vi "GUI_OpticalSpectromete_oldr.vi"() -> ()   [LabVIEW 2009]
uses:
  shared programs/sentCommandSetting.vi
panel:
  out "new D Data":bool=TRUE
  out "new S Data":bool
  out "new Slow Data":bool=TRUE
  out "error out 5":errorcluster
  out "new Device Data":bool=TRUE
  in  "Tab Control 2":enum32{"debug", "plain", "plain 2"}(tab)
  out "message from device":string
  out "data out 2":string
  out "error out 3":errorcluster
  in  "after substring":string="-0.089798,-0.012312,-0.023161,-0.029413,-0.099722,-0.082148,-0.175780,-0.016640,-0.021793,-0.106872,-0.083723,0.034795,-0.021191,0.038109,0.089728,0.030656,0.190136,0.095931,0.069651,0.042030,-0.035811,-0.039992,-0.152535,-0.081980,-0.239391,-0.299099,-0.220282,-0.102308,-0.243030,-0.071880,-0.064330,0.057168,0.183804,0.430142,0.593920,0.668964,0.765233,0.852774,1.014855,0.897499,1.075418,0.964040,0.859461,0.844898,0.817245,0.729092,0.485039,0.430748,0.147230,0.101254,-0.023353,0.001419,-0.101078,-0.215137,-0.151236,-0.187878,-0.201514,-0.145757,-0.076726,-0.030284,0.027449,0.054593,0.122555,0.149751,0.201496,0.172129,0.177528,0.053173,0.056690,-0.060797,-0.012635,-0.050433,-0.055065,-0.118074,-0.067874,-0.150187,-0.037475,-0.162903,0.037664,-0.067378,0.033191,0.067444,0.129342,0.131002,0.036134,0.129384,0.095361,0.030507,0.046942,-0.075844,-0.066935,0.066320,-0.017437,0.050973,-0.012719,-0.028872,-0.007972,-0.092477,-0.020650,-0.016307\r\n"
  in  "command 3":string="1Darray"
  in  "after substring 3":string
  out "settings 2":string[][](array[string])=[["no error", ">>on"]]
  in  "data out 3":string="Spectrometer>>1Darray>>-0.089798,-0.012312,-0.023161,-0.029413,-0.099722,-0.082148,-0.175780,-0.016640,-0.021793,-0.106872,-0.083723,0.034795,-0.021191,0.038109,0.089728,0.030656,0.190136,0.095931,0.069651,0.042030,-0.035811,-0.039992,-0.152535,-0.081980,-0.239391,-0.299099,-0.220282,-0.102308,-0.243030,-0.071880,-0.064330,0.057168,0.183804,0.430142,0.593920,0.668964,0.765233,0.852774,1.014855,0.897499,1.075418,0.964040,0.859461,0.844898,0.817245,0.729092,0.485039,0.430748,0.147230,0.101254,-0.023353,0.001419,-0.101078,-0.215137,-0.151236,-0.187878,-0.201514,-0.145757,-0.076726,-0.030284,0.027449,0.054593,0.122555,0.149751,0.201496,0.172129,0.177528,0.053173,0.056690,-0.060797,-0.012635,-0.050433,-0.055065,-0.118074,-0.067874,-0.150187,-0.037475,-0.162903,0.037664,-0.067378,0.033191,0.067444,0.129342,0.131002,0.036134,0.129384,0.095361,0.030507,0.046942,-0.075844,-0.066935,0.066320,-0.017437,0.050973,-0.012719,-0.028872,-0.007972,-0.092477,-0.020650,-0.016307\r\n"
  out "after substring 2":string="no error,>>on"
  out "device ID":refnum<k16>
  in  "Tab Control":enum32{"Main", "Network settings", "internal"}(tab)
  in  "getSettings":bool
  in  "setTrigger":bool
  in  "String":string="subscribe>>opticalspectrometer"
  in  "sent":bool
  in  "setSave":bool
  out "save":bool
  in  "setExposure":dbl=2.0
  out "exposure out":dbl=2.0
  out "value":string
  out "trigger":bool
  out "array 2":dbl[](graph)=[-0.089798, -0.012312, -0.023161, -0.029413, -0.099722, -0.082148, -0.17578, -0.01664, -0.021793, -0.106872, -0.083723, 0.034795, -0.021191, 0.038109, 0.089728, 0.030656, 0.190136, 0.095931, 0.069651, 0.04203, -0.035811, -0.039992, -0.152535, -0.08198, -0.239391, -0.299099, -0.220282, -0.102308, -0.24303, -0.07188, -0.06433, 0.057168, 0.183804, 0.430142, 0.59392, 0.668964, 0.765233, 0.852774, 1.014855, 0.897499, 1.075418, 0.96404, 0.859461, 0.844898, 0.817245, 0.729092, 0.485039, 0.430748, 0.14723, 0.101254, -0.023353, 0.001419, -0.101078, -0.215137, -0.151236, -0.187878, -0.201514, -0.145757, -0.076726, -0.030284, 0.027449, 0.054593, 0.122555, 0.149751, 0.201496, 0.172129, 0.177528, 0.053173, 0.05669, -0.060797, -0.012635, -0.050433, -0.055065, -0.118074, -0.067874, -0.150187, -0.037475, -0.162903, 0.037664, -0.067378, 0.033191, 0.067444, 0.129342, 0.131002, 0.036134, 0.129384, 0.095361, 0.030507, 0.046942, -0.075844, -0.066935, 0.06632, -0.017437, 0.050973, -0.012719, -0.028872, -0.007972, -0.092477, -0.02065, -0.016307]
  in  "local Port":u16=61557
  in  "Remote Host":string="192.168.10.156"
  in  "port or service name":u16=65525
  in  "timeout ms (100)":i32=500
  out "fast ID":refnum<k16>
  out "slow ID":refnum<k16>
  out "error out":errorcluster
  out "Image Pixels (U8) 5":u8[][](graph)
  in  "stop":bool
  # "61525"
  # "65535"
  # "61533"
  # "localhost"
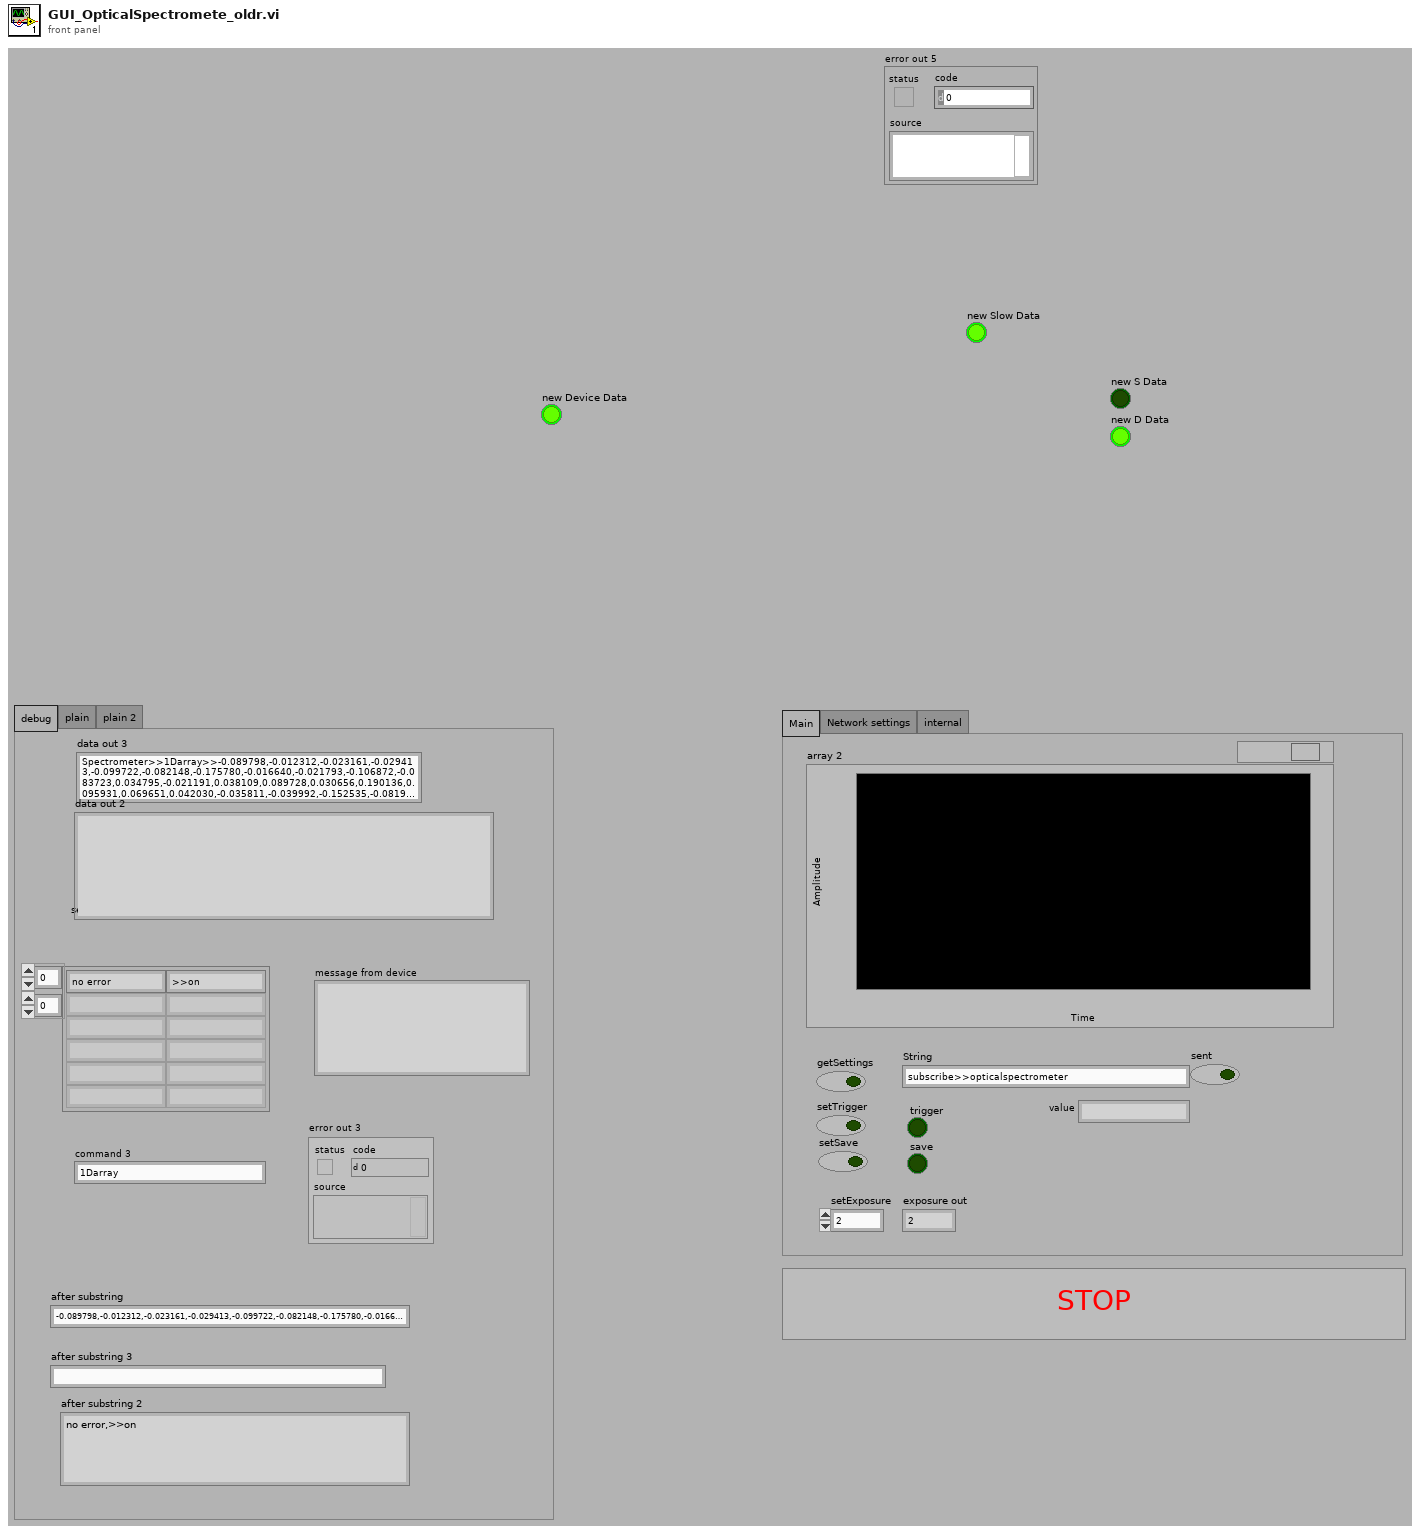
[diagram p1: front panel]
types:
  T1 = typedef "Image Type" = u32
  T2 = typedef "IMAQ Image.ctl" = refnum<image>
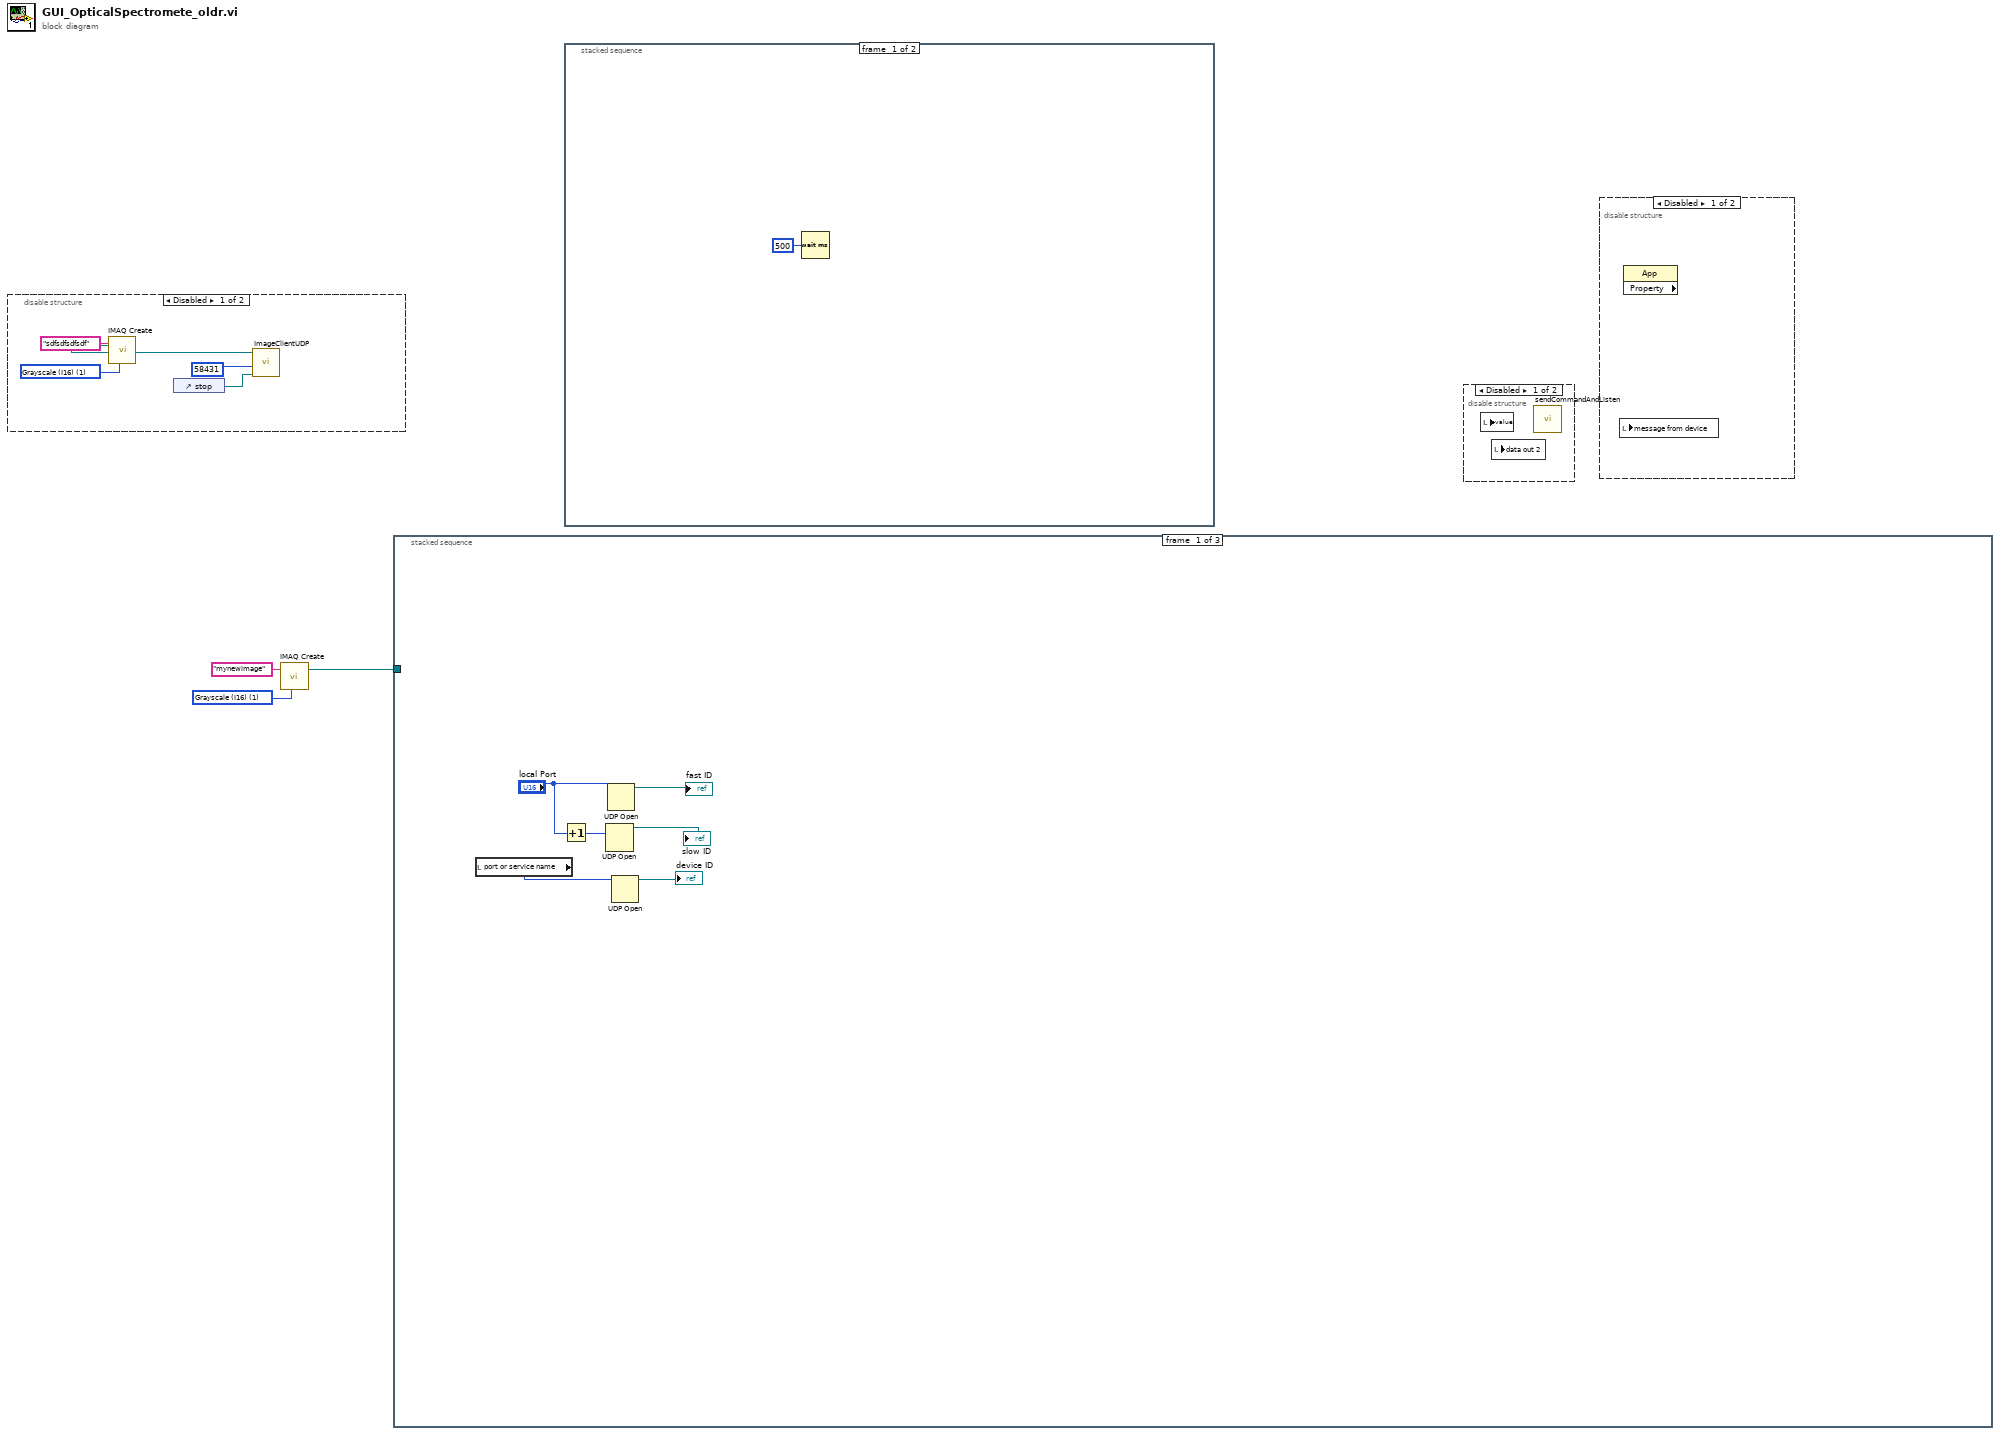
[diagram p0: block diagram]
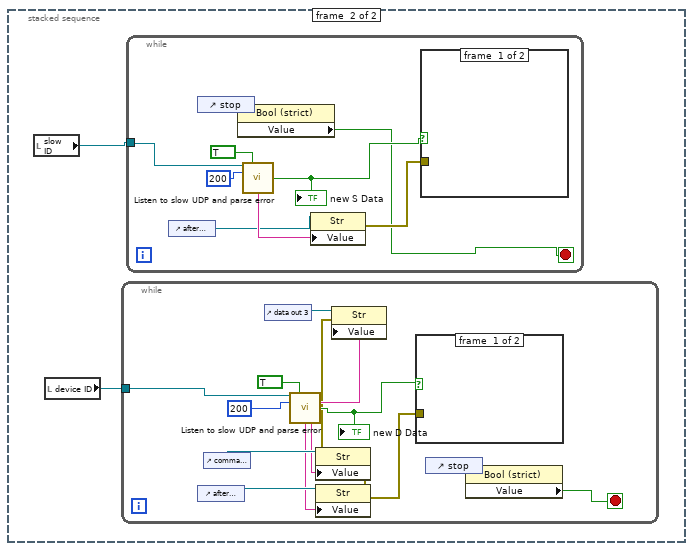
[diagram p2: hidden frame]
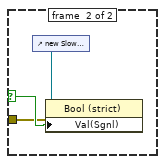
[diagram p3: hidden frame]
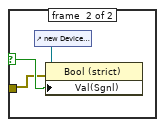
[diagram p4: hidden frame]
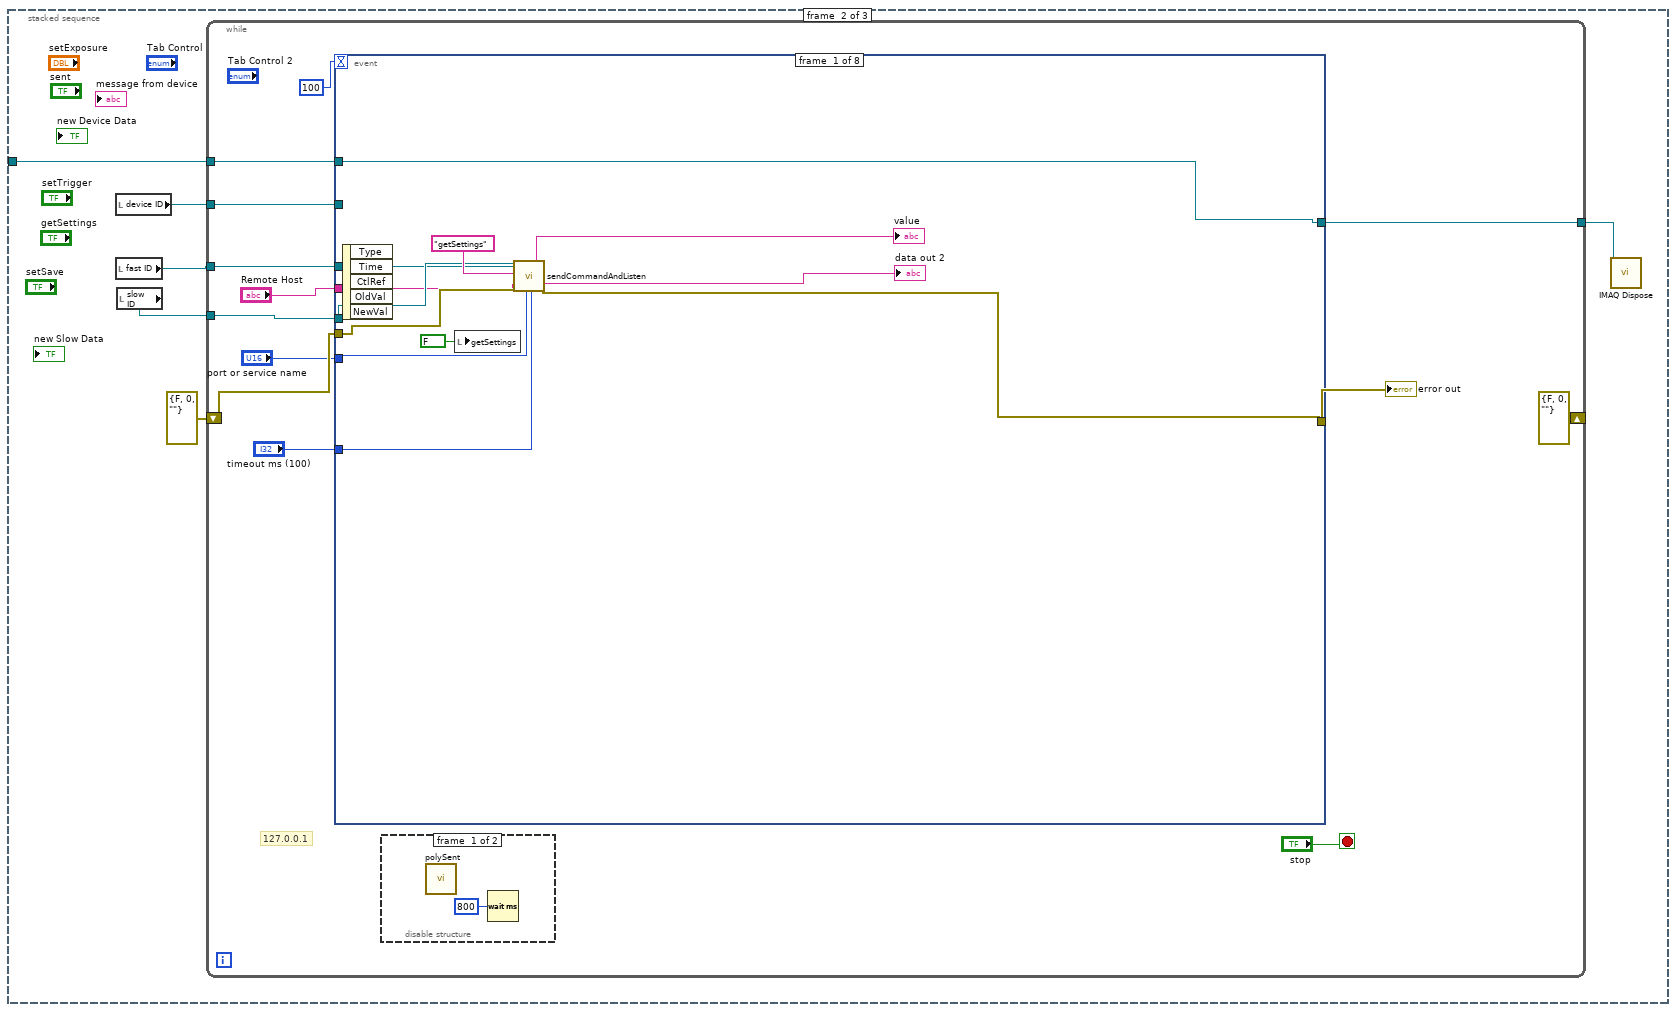
[diagram p8: hidden frame]
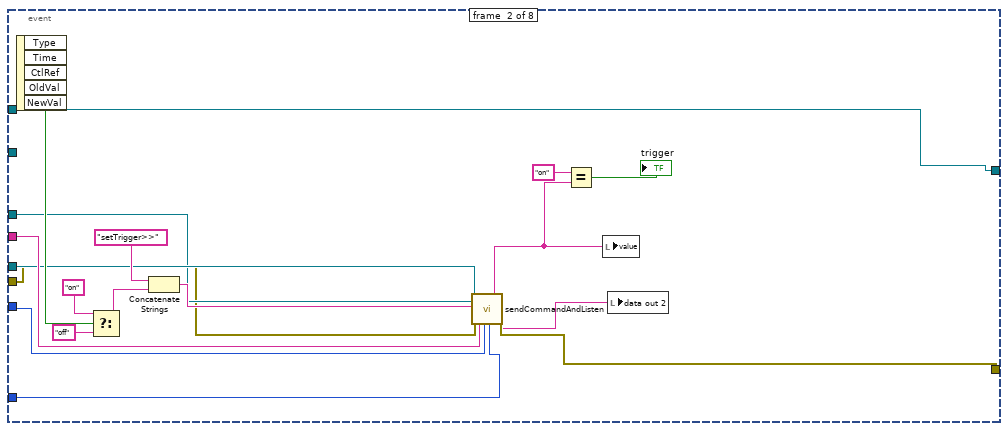
[diagram p9: hidden frame]
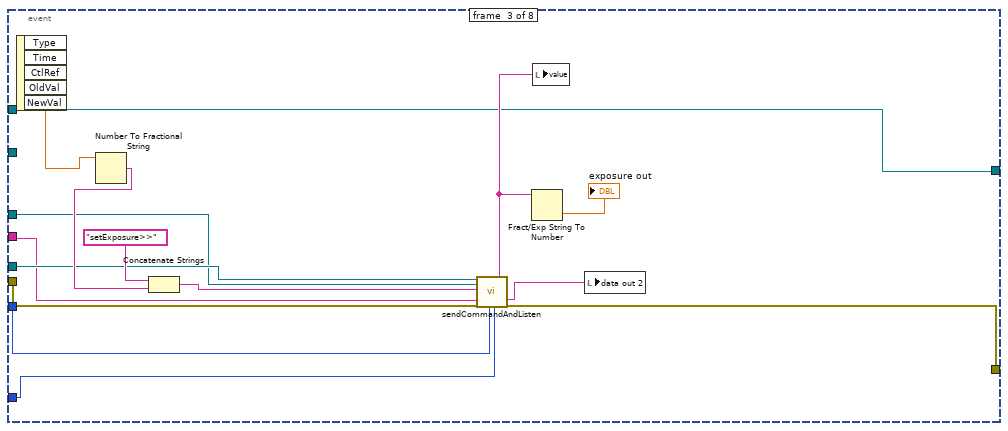
[diagram p10: hidden frame]
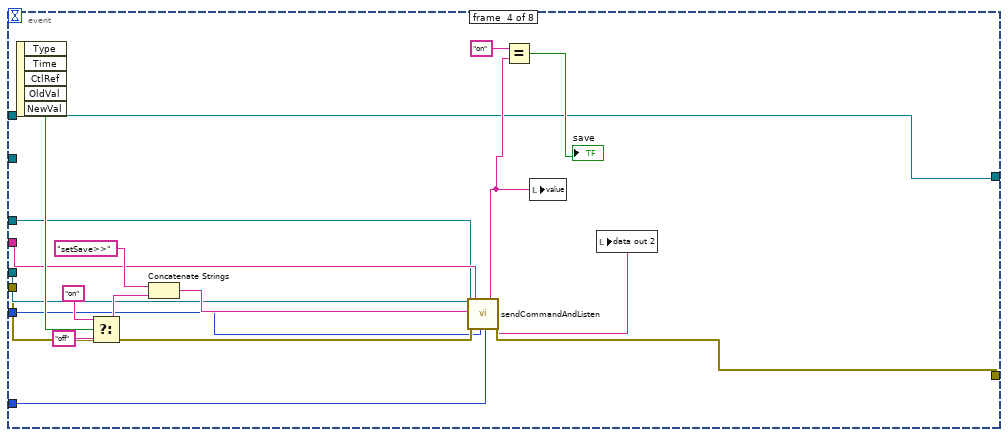
[diagram p11: hidden frame]
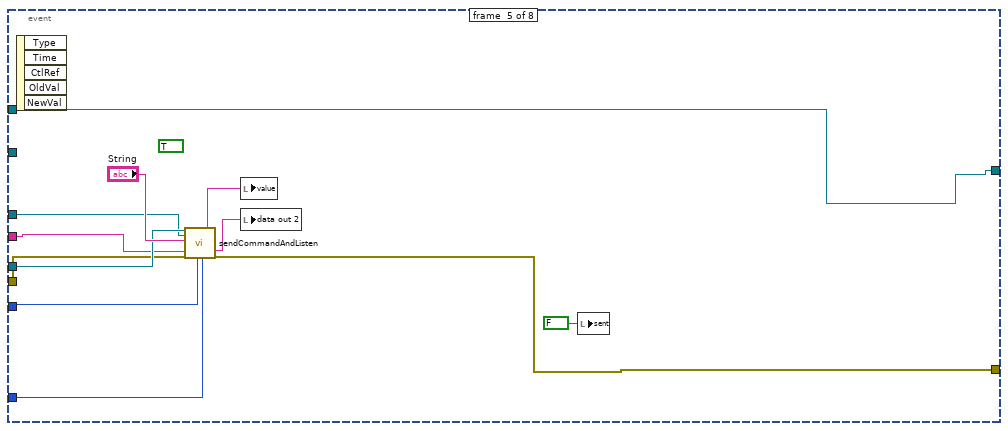
[diagram p12: hidden frame]
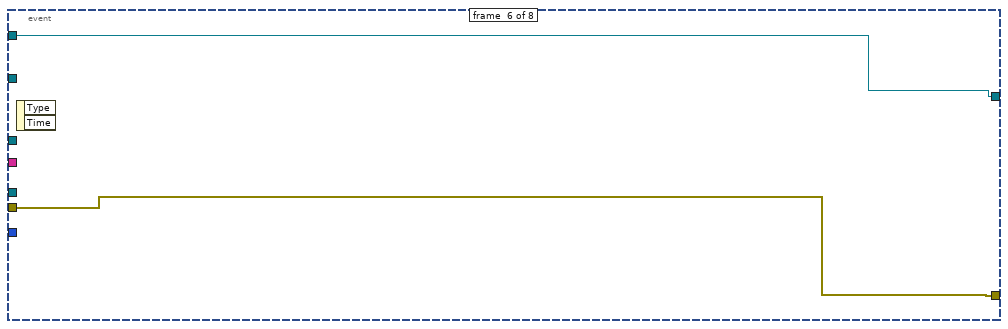
[diagram p13: hidden frame]
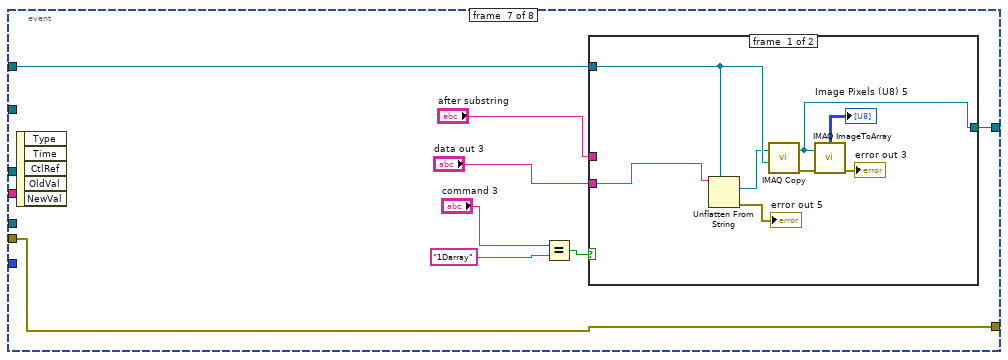
[diagram p14: hidden frame]
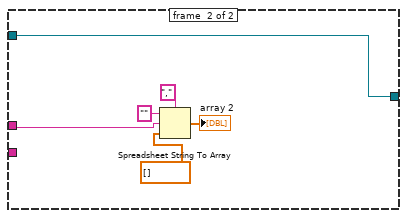
[diagram p15: hidden frame]
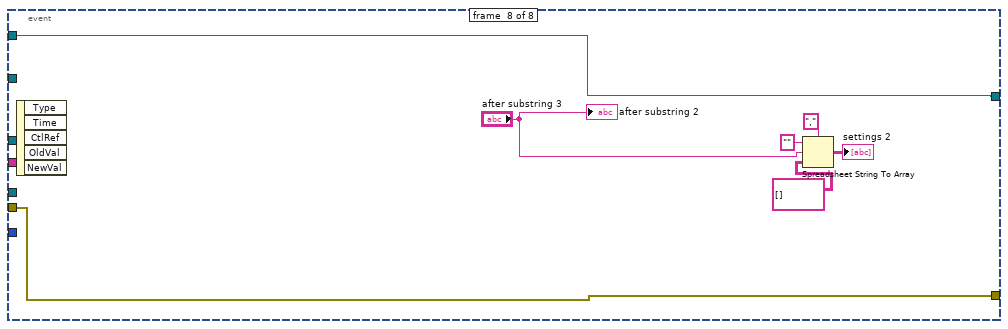
[diagram p16: hidden frame]
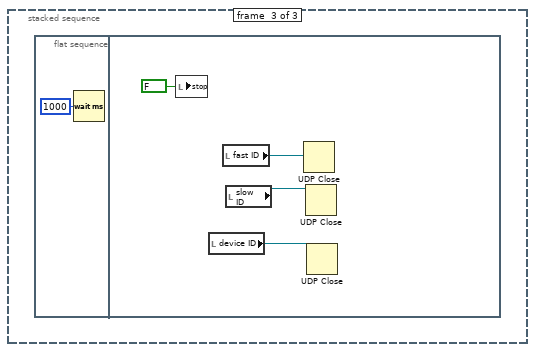
[diagram p18: hidden frame]
diagram:
  w3 = T1 1 items=["Grayscale (U8)", "Grayscale (I16)", "Grayscale (SGL)", "Complex (CSG)", "RGB (U32)", "HSL (U32)", "RGB (U64)", "Grayscale (U16)"] ("Image Type")
  n1 = disable-structure shown="Disabled" {
    frame #0 {
      w6 = T1 1 items=["Grayscale (U8)", "Grayscale (I16)", "Grayscale (SGL)", "Complex (CSG)", "RGB (U32)", "HSL (U32)", "RGB (U64)", "Grayscale (U16)"] ("Image Type")
      n2 = call "IMAQ Create"("Image Name"="sdfsdfsdfsdf", "Image Type"=w6) -> ("New Image"=w4:T2)  [unwired: 3 in, 1 out]
      n3 = control-ref of="stop"() -> (w11:refnum<vi>)
      n4 = call "ImageClientUDP.vi"("Stop 2"=w11, "image port"=58431, "New Image"=w4) -> ("Image Pixels (U8) 4"=w9:refnum<vi>, "TIME"=w7:refnum<vi>, "connected 2"=w8:refnum<vi>)  [unwired: 5 in, 1 out]
    }
    frame #1 {
    }
  }
  n5 = call "IMAQ Create"("Image Name"="mynewimage", "Image Type"=w3) -> ("New Image"=w1:T2)  [unwired: 3 in, 1 out]
  n6 = stacked-sequence {
    tunnel: w1 -> [_ w20 _]
    frame #0 {
      n7 = local read "port or service name"() -> (w13:u16)
      n8 = Increment(x="local Port") -> (x+1=w15:u16)
      n9 = UDP Open(11:w15) -> (port=→"slow ID":refnum<k16>)  [unwired: 4 in, 2 out]
      n10 = UDP Open(11:"local Port") -> (port=→"fast ID":refnum<k16>)  [unwired: 4 in, 2 out]
      n11 = UDP Open(11:w13) -> (port=→"device ID":refnum<k16>)  [unwired: 4 in, 2 out]
    }
    frame #1 {
      n12 = local read "device ID"() -> (w18:refnum<k16>)
      n13 = local read "fast ID"() -> (w22:refnum<k16>)
      n14 = local read "slow ID"() -> (w21:refnum<k16>)
      n15 = while {
        tunnel: w22 -> [w35]
        shift-right: [errorcluster {"status"=FALSE, "code"=0, "source"=""} ("error out")] -> _
        shift-left: errorcluster {"status"=FALSE, "code"=0, "source"=""} ("error out") -> [w33]
        tunnel: w21 -> [w27]
        tunnel: w20 -> [w26]
        tunnel: [w25] -> w19
        tunnel: w18 -> [w24]
        stop <- "stop" stop-if-true
        # "127.0.0.1"
        n16 = event shown="[6] \"new Device Data \": Value Change" {
          selector: _ -> [_ _ _ _ _ _ _ _]
          dyn-events: _ -> [_ _ _ _ _ _ _ _]
          timeout: 100 -> [_ _ _ _ _ _ _ _]
          tunnel: w35 -> [w45 w56 w76 w92 w108 _ _ _]
          tunnel: [w43 w54 w74 w89 w106 w112 w116 w142] -> w34
          tunnel: w33 -> [w44 w55 w75 w90 w107 w112 w116 w142]
          tunnel: "Remote Host" -> [w42 w59 w72 w93 w105 _ _ _]
          tunnel: "port or service name" -> [w41 w60 w71 w88 w104 _ _ _]
          tunnel: "timeout ms (100)" -> [w40 w61 w70 w87 w103 _ _ _]
          tunnel: w27 -> [w46 w57 w77 w91 w109 _ _ _]
          tunnel: w26 -> [w37 w49 w67 w82 w100 w113 w121 w140]
          tunnel: [w37 w49 w67 w82 w100 w113 w120 w140] -> w25
          tunnel: w24 -> [_ _ _ _ _ _ _ _]
          event #0 {
            n17 = event-data() -> ()  [unwired: 1 in, 5 out]
            n18 = local write "getSettings"(FALSE ("getSettings")) -> ()
            n19 = call "sendCommandAndListen.vi"("ID slow"=w46, "ID fast"=w45, "command in"="getSettings" ("data in"), "error in"=w44, "Remote Host"=w42, "port or service name"=w41, "timeout ms (100)"=w40) -> ("value"=→"value":string, "data out"=→"data out 2":string, "error out"=w43:errorcluster)  [unwired: 7 in, 3 out]
          }
          event #1 {
            n20 = event-data() -> ("NewVal"=w66:bool)  [unwired: 1 in, 4 out]
            n21 = Select(t="on", s=w66, f="off") -> (s? t:f=w62:string)
            n22 = Concatenate Strings("setTrigger>>" ("data in"), w62) -> (w58:string)
            n23 = call "sendCommandAndListen.vi"("ID slow"=w57, "ID fast"=w56, "command in"=w58, "error in"=w55, "Remote Host"=w59, "port or service name"=w60, "timeout ms (100)"=w61) -> ("value"=w51:string, "data out"=w53:string, "error out"=w54:errorcluster)  [unwired: 7 in, 3 out]
            n24 = Equal?(x="on", y=w51) -> (x = y?=→"trigger":bool)
            n25 = local write "value"(w51) -> ()
            n26 = local write "data out 2"(w53) -> ()
          }
          event #2 {
            n27 = event-data() -> ("NewVal"=w79:dbl)  [unwired: 1 in, 4 out]
            n28 = Number To Fractional String(number=w79) -> (F-format string=w80:string)  [unwired: 3 in]
            n29 = Concatenate Strings("setExposure>>" ("data in"), w80) -> (w78:string)
            n30 = call "sendCommandAndListen.vi"("ID slow"=w77, "ID fast"=w76, "command in"=w78, "error in"=w75, "Remote Host"=w72, "port or service name"=w71, "timeout ms (100)"=w70) -> ("value"=w69:string, "data out"=w73:string, "error out"=w74:errorcluster)  [unwired: 7 in, 3 out]
            n31 = Fract/Exp String To Number(string=w69) -> (number=→"exposure out":dbl)  [unwired: 3 in, 1 out]
            n32 = local write "value"(w69) -> ()
            n33 = local write "data out 2"(w73) -> ()
          }
          event #3 {
            n34 = event-data() -> ("NewVal"=w99:bool)  [unwired: 1 in, 4 out]
            n35 = Select(t="on", s=w99, f="off") -> (s? t:f=w95:string)
            n36 = Concatenate Strings("setSave>>" ("data in"), w95) -> (w94:string)
            n37 = call "sendCommandAndListen.vi"("ID slow"=w91, "ID fast"=w92, "command in"=w94, "error in"=w90, "Remote Host"=w93, "port or service name"=w88, "timeout ms (100)"=w87) -> ("value"=w85:string, "data out"=w86:string, "error out"=w89:errorcluster)  [unwired: 7 in, 3 out]
            n38 = Equal?(x="on", y=w85) -> (x = y?=→"save":bool)
            n39 = local write "value"(w85) -> ()
            n40 = local write "data out 2"(w86) -> ()
          }
          event #4 {
            (unwired) TRUE ("Boolean")
            n41 = event-data() -> ()  [unwired: 1 in, 5 out]
            n42 = call "sendCommandAndListen.vi"("ID slow"=w109, "ID fast"=w108, "command in"="String", "error in"=w107, "Remote Host"=w105, "port or service name"=w104, "timeout ms (100)"=w103) -> ("value"=w101:string, "data out"=w102:string, "error out"=w106:errorcluster)  [unwired: 7 in, 3 out]
            n43 = local write "value"(w101) -> ()
            n44 = local write "data out 2"(w102) -> ()
            n45 = local write "sent"(FALSE ("sent")) -> ()
          }
          event #5 {
            n46 = event-data() -> ()  [unwired: 1 in, 2 out]
          }
          event #6 {
            n47 = event-data() -> ()  [unwired: 1 in, 5 out]
            n48 = Equal?(x="command 3", y="1Darray") -> (x = y?=w114:bool)
            n49 = case shown="True" w114 {
              tunnel: "after substring" -> [_ w135]
              tunnel: w121 -> [w129 w130]
              tunnel: [w128 w130] -> w120
              tunnel: "data out 3" -> [w127 _]
              frame #0 {
                n50 = Unflatten From String(type=w129, binary string=w127) -> (value=w126:T2, error out=→"error out 5":errorcluster)  [unwired: 1 in, 3 out]
                n51 = call "IMAQ Copy"("Image Dst"=w129, "Image Src"=w126) -> ("error out"=w124:errorcluster, "Image Dst Out"=w128:T2)  [unwired: 4 in]
                n52 = call "IMAQ ImageToArray"("error in (no error)"=w124, "Image"=w128) -> ("error out"=→"error out 3":errorcluster, "Image Pixels (U8)"=→"Image Pixels (U8) 5":u8[][])  [unwired: 2 in, 3 out]
              }
              frame #1 {
                n53 = Spreadsheet String To Array(delimiter (Tab)=",", format string="", spreadsheet string=w135, array type (2D Dbl)=dbl[] []) -> (array=→"array 2":dbl[])
              }
            }
          }
          event #7 {
            n54 = event-data() -> ()  [unwired: 1 in, 5 out]
            n55 = Spreadsheet String To Array(delimiter (Tab)=",", format string="", spreadsheet string="after substring 3", array type (2D Dbl)=string[][] []) -> (array=→"settings 2":string[][])
            "after substring 2" <- "after substring 3"
          }
        }
        "error out" <- w34
        n56 = disable-structure shown="Enabled" {
          frame #0 {
            n57 = call-poly "polySent.vi"() -> ()  [unwired: 11 in]
            n58 = Wait (ms)(milliseconds to wait=u32 800) -> ()  [unwired: 1 out]
          }
          frame #1 {
          }
        }
      }
      n59 = call "IMAQ Dispose"("Image"=w19) -> ()  [unwired: 5 in, 1 out]
    }
    frame #2 {
      n60 = flat-sequence {
        frame #0 {
          n61 = Wait (ms)(milliseconds to wait=u32 1000) -> ()  [unwired: 1 out]
        }
        frame #1 {
          n62 = local write "stop"(FALSE ("stop")) -> ()
          n63 = local read "device ID"() -> (w145:refnum<k16>)
          n64 = local read "fast ID"() -> (w146:refnum<k16>)
          n65 = local read "slow ID"() -> (w147:refnum<k16>)
          n66 = UDP Close(connection ID=w146) -> ()  [unwired: 1 in, 2 out]
          n67 = UDP Close(connection ID=w147) -> ()  [unwired: 1 in, 2 out]
          n68 = UDP Close(connection ID=w145) -> ()  [unwired: 1 in, 2 out]
        }
      }
    }
  }
  n69 = stacked-sequence {
    frame #0 {
      n70 = Wait (ms)(milliseconds to wait=u32 500) -> ()  [unwired: 1 out]
    }
    frame #1 {
      n71 = local read "slow ID"() -> (w150:refnum<k16>)
      n72 = local read "device ID"() -> (w151:refnum<k16>)
      n73 = while {
        tunnel: w151 -> [w176]
        stop <- w164 stop-if-true
        n74 = control-ref of="after substring"() -> (w170:refnum<vi>)
        n75 = control-ref of="command 3"() -> (w172:refnum<vi>)
        n76 = control-ref of="data out 3"() -> (w174:refnum<vi>)
        n77 = call "Listen to slow UDP and parse error.vi"("ID slow"=w176, "command accepted"=TRUE, "timeout ms (25000)"=200) -> ("data out"=w173:string, "new Data"=w175:bool, "after substring"=w169:string, "command"=w171:string)  [unwired: 5 in, 4 out]
        "new D Data" <- w175
        n78 = property class="Str"(reference=w174, "Value"=w173) -> (error out=w168:errorcluster)  [unwired: 1 in, 1 out]
        n79 = property class="Str"(reference=w172, error in=w168, "Value"=w171) -> (error out=w167:errorcluster)  [unwired: 1 out]
        n80 = property class="Str"(reference=w170, error in=w167, "Value"=w169) -> (error out=w166:errorcluster)  [unwired: 1 out]
        n81 = case shown="True" w175 {
          selector: w175 -> [_ w181]
          tunnel: w166 -> [_ w179]
          frame #0 {
          }
          frame #1 {
            n82 = control-ref of="new Device Data"() -> (w180:refnum<vi>)
            n83 = property class="Bool (strict)"(reference=w180, error in=w179, "Val(Sgnl)"=w181) -> ()  [unwired: 2 out]
          }
        }
        n84 = control-ref of="stop"() -> (w165:refnum<vi>)
        n85 = property class="Bool (strict)"(reference=w165) -> ("Value"=w164:bool)  [unwired: 1 in, 2 out]
      }
      n86 = while {
        tunnel: w150 -> [w158]
        stop <- w152 stop-if-true
        n87 = control-ref of="after substring 3"() -> (w155:refnum<vi>)
        n88 = control-ref of="stop"() -> (w153:refnum<vi>)
        n89 = property class="Bool (strict)"(reference=w153) -> ("Value"=w152:bool)  [unwired: 1 in, 2 out]
        n90 = call "Listen to slow UDP and parse error.vi"("ID slow"=w158, "command accepted"=TRUE, "timeout ms (25000)"=200) -> ("new Data"=w157:bool, "after substring"=w156:string)  [unwired: 5 in, 6 out]
        "new S Data" <- w157
        n91 = property class="Str"(reference=w155, "Value"=w156) -> (error out=w154:errorcluster)  [unwired: 1 in, 1 out]
        n92 = case shown="True" w157 {
          selector: w157 -> [_ w163]
          tunnel: w154 -> [_ w161]
          frame #0 {
          }
          frame #1 {
            n93 = control-ref of="new Slow Data"() -> (w162:refnum<vi>)
            n94 = property class="Bool (strict)"(reference=w162, error in=w161, "Val(Sgnl)"=w163) -> ()  [unwired: 2 out]
          }
        }
      }
    }
  }
  n95 = disable-structure shown="Disabled" {
    frame #0 {
      n96 = local read "value"() -> ()  [unwired: 1 in]
      n97 = local read "data out 2"() -> ()  [unwired: 1 in]
      n98 = call "sendCommandAndListen.vi"() -> ()  [unwired: 14 in, 6 out]
    }
    frame #1 {
    }
  }
  n99 = disable-structure shown="Disabled" {
    frame #0 {
      n100 = local read "message from device"() -> ()  [unwired: 1 in]
      n101 = property class="App" props=[]() -> ()  [unwired: 2 in, 3 out]
    }
    frame #1 {
    }
  }
